vi "RT Stop.vi"() -> ()   [LabVIEW 2016]
panel:
  in  "I/O loop running":bool
  in  "serial loop running":bool
  in  "serial port output enabled?":bool
  in  "RT Stop":bool
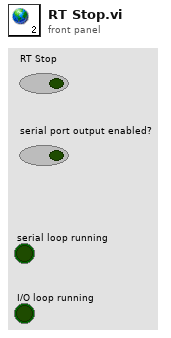
[diagram p1: front panel]
diagram:
